vi "Write FQN (T).vi"(8 "error in (no error)":errorcluster, 10 "FQN (T)":bool=TRUE, 11 "Class Loader in":refnum<class "Class Loader.lvclass">) -> (0 "error out":errorcluster, 3 "Class Loader out":refnum<class "Class Loader.lvclass">)   [LabVIEW 2023, in "Class Loader.lvlib" / "Class Loader.lvclass"]
uses:
  Class Loader.lvclass
  Class Loader.lvclass/Class Loader.ctl
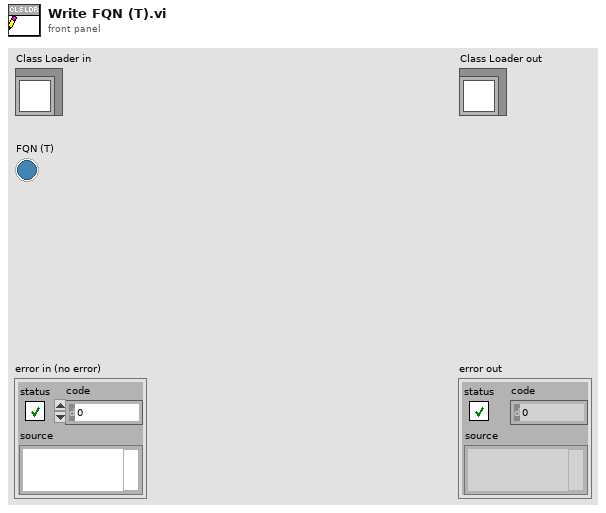
[diagram p1: front panel]
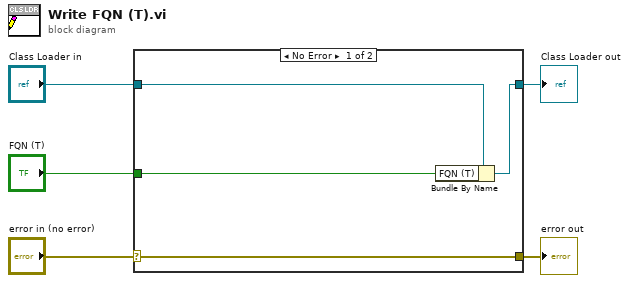
[diagram p0: block diagram]
diagram:
  n1 = case shown="No Error" "error in (no error)" {
    selector: "error in (no error)" -> [w9 w10]
    tunnel: [w9 w10] -> w4
    tunnel: [w7 w11] -> w2
    tunnel: "Class Loader in" -> [w8 w11]
    tunnel: "FQN (T)" -> [w6 _]
    frame No Error {
      n2 = Bundle By Name(cluster=w8, "FQN (T)"=w6) -> (w7:refnum<class "Class Loader.lvclass">)
    }
    frame Error {
    }
  }
  "error out" <- w4
  "Class Loader out" <- w2
